vi "TcA04-002_ForceParentCallMethods.vi"(1 "Input buffer":T3="1", 3 "Invocation info":T2, 5 "error in (no error)":errorcluster, 6 "Add log to result?":bool) -> (16 "Test Data":T1 {"Numeric Measurement" format="%.2f"}, 19 "error out":errorcluster)   [LabVIEW 2020]
doc: "Test case template."
uses:
  Shared/Support_InputBuffer.ctl
  Shared/Support_InvocationInfo.ctl
  Shared/Support_TestData.ctl
  TestClasses/G#BaseClass1_class/G#BaseClass1.lvclass
  TestClasses/G#SubClass1_class/G#SubClass1.lvclass
  C:/Program Files (x86)/National Instruments/LabVIEW 2020/vi.lib/addons/_AddQ/G#Object/G#Object.lvclass
  TestClasses/G#SubSubClass1_class/G#SubSubClass1.lvclass
  <vilib>/addons/_AddQ/G#Object/G#Object.lvclass
panel:
  in  "Test name":string="TcA04-002 Force Parent Call Methods"
  out "Test result":bool
  out "Result":string
  # "Verify that a sub class method can be dynamically called\n(if there exists one) by a virtually declared base \nclass method else base class implementation is used."
  # "Sub test case"
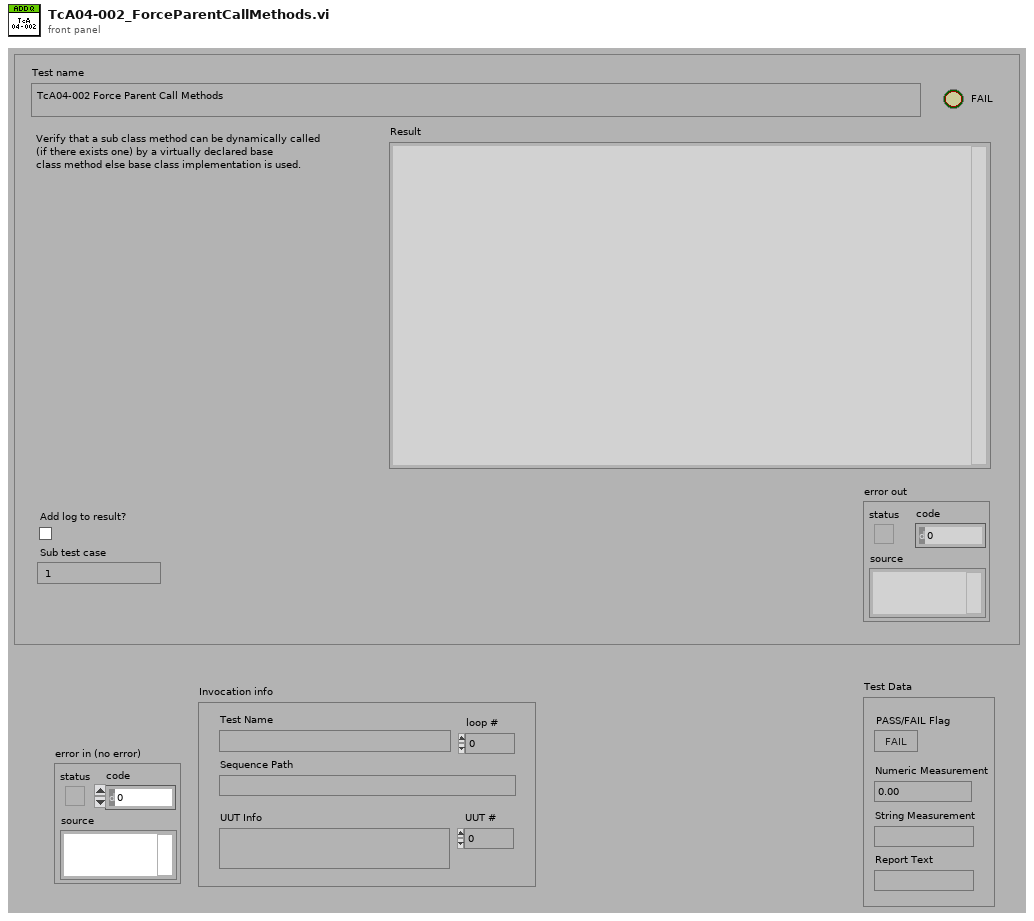
[diagram p1: front panel]
types:
  T1 = typedef "Support_TestData.ctl" = cluster{"PASS/FAIL Flag":bool, "Numeric Measurement":dbl, "String Measurement":string, "Report Text":string}
  T2 = typedef "Support_InvocationInfo.ctl" = cluster{"UUT #":i32, "loop #":i32, "UUT Info":string, "Test Name":string, "Sequence Path":path}
  T3 = typedef "Support_InputBuffer.ctl" = string
  T4 = typedef "Support_ResultType.ctl" = cluster{"Pass":bool, "Comment":string, "MeasurementValue":dbl}
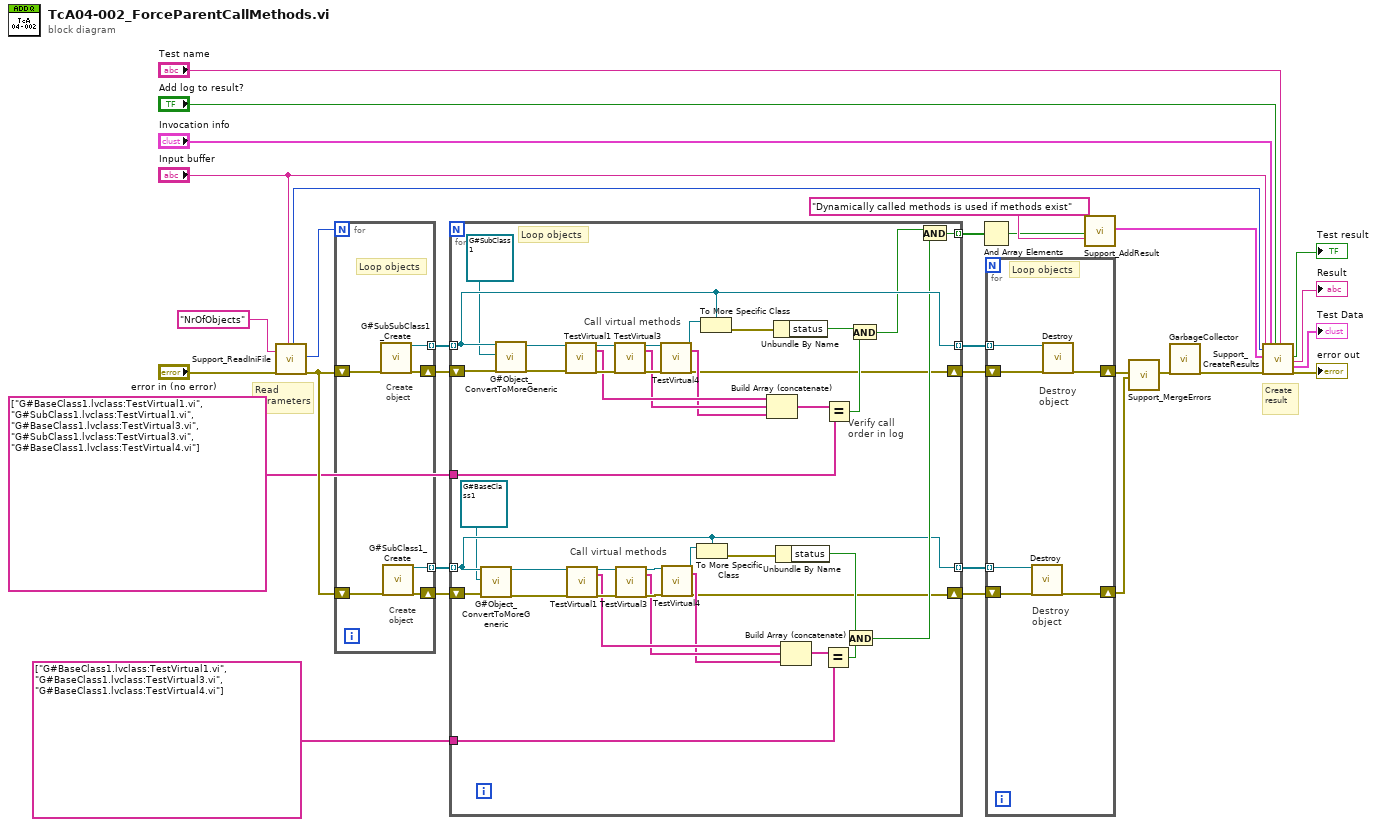
[diagram p0: block diagram]
diagram:
  # "Create\nresult"
  # "Read\nparameters"
  n1 = call "Support_ReadIniFile.vi"("Parameter name"="NrOfObjects", "error in (no error)"="error in (no error)", "Sub test case"="Input buffer") -> ("Timer start"=w21:u32, "Parameter1 as I32"=w18:i32, "error out"=w8:errorcluster)  [unwired: 9 in, 5 out]
  n2 = for {
    N: w18 -> [_]
    tunnel: [w37] -> w15 mode=indexing
    shift-right: [w36] -> w16
    shift-left: w8 -> [w35]
    shift-right: [w33] -> w6
    shift-left: w8 -> [w34]
    tunnel: [w32] -> w7 mode=indexing
    # "Create\nobject"
    # "Loop objects"
    # "Create\nobject"
    n3 = call "G#SubSubClass1_Create.vi"("error in (no error)"=w35) -> ("reference out"=w37:refnum<class "G#SubSubClass1.lvclass">, "error out"=w36:errorcluster)  [unwired: 17 in]
    n4 = call "G#SubClass1_Create.vi"("error in (no error)"=w34) -> ("reference out"=w32:refnum<class "G#SubClass1.lvclass">, "error out"=w33:errorcluster)  [unwired: 16 in, 1 out]
  }
  n5 = for {
    shift-right: [w41] -> w14
    shift-left: w16 -> [w57]
    tunnel: w15 -> [w56] mode=indexing
    tunnel: [w56] -> w13 mode=indexing
    tunnel: [w78] -> w12 mode=indexing
    tunnel: w7 -> [w44] mode=indexing
    shift-right: [w40] -> w4
    shift-left: w6 -> [w45]
    tunnel: [w44] -> w5 mode=indexing
    tunnel: string[] ["G#BaseClass1.lvclass:TestVirtual1.vi", "G#SubClass1.lvclass:TestVirtual1.vi", "G#BaseClass1.lvclass:TestVirtual3.vi", "G#SubClass1.lvclass:TestVirtual3.vi", "G#BaseClass1.lvclass:TestVirtual4.vi"] ("appended array") -> [w60]
    tunnel: string[] ["G#BaseClass1.lvclass:TestVirtual1.vi", "G#BaseClass1.lvclass:TestVirtual3.vi", "G#BaseClass1.lvclass:TestVirtual4.vi"] ("appended array 2") -> [w58]
    # "Call virtual methods"
    # "Call virtual methods"
    # "Loop objects"
    # "Verify call\norder in log"
    n6 = call-dynamic "G#Object_ConvertToMoreGeneric.vi"("reference in"=w44, "convert to"=refnum<class "G#BaseClass1.lvclass"> refnum ("G#BaseClass1.lvclass"), "error in (no error)"=w45) -> ("converted reference out"=w42:refnum<class "G#BaseClass1.lvclass">, "error out"=w43:errorcluster)  [unwired: 15 in]
    n7 = call-dynamic "G#Object_ConvertToMoreGeneric.vi"("reference in"=w56, "convert to"=refnum<class "G#SubClass1.lvclass"> refnum ("G#SubClass1.lvclass"), "error in (no error)"=w57) -> ("converted reference out"=w54:refnum<class "G#SubClass1.lvclass">, "error out"=w55:errorcluster)  [unwired: 15 in]
    n8 = call-dynamic "TestVirtual1.vi"("reference in"=w54, "error in (no error)"=w55) -> ("reference out"=w75:refnum<class "G#SubClass1.lvclass">, "MethodName"=w67:string[], "error out"=w77:errorcluster)  [unwired: 15 in]
    n9 = call-dynamic "TestVirtual1.vi"("reference in"=w42, "error in (no error)"=w43) -> ("reference out"=w71:refnum<class "G#BaseClass1.lvclass">, "MethodName"=w63:string[], "error out"=w70:errorcluster)  [unwired: 15 in]
    n10 = call-dynamic "TestVirtual3.vi"("reference in"=w75, "error in (no error)"=w77) -> ("reference out"=w74:refnum<class "G#SubClass1.lvclass">, "MethodName"=w66:string[], "error out"=w76:errorcluster)  [unwired: 15 in]
    n11 = call-dynamic "TestVirtual3.vi"("reference in"=w71, "error in (no error)"=w70) -> ("reference out"=w72:refnum<class "G#BaseClass1.lvclass">, "MethodName"=w62:string[], "error out"=w69:errorcluster)  [unwired: 15 in]
    n12 = call-dynamic "TestVirtual4.vi"("reference in"=w74, "error in (no error)"=w76) -> ("reference out"=w73:refnum<class "G#SubClass1.lvclass">, "MethodName"=w65:string[], "error out"=w41:errorcluster)  [unwired: 15 in]
    n13 = call-dynamic "TestVirtual4.vi"("reference in"=w72, "error in (no error)"=w69) -> ("reference out"=w68:refnum<class "G#BaseClass1.lvclass">, "MethodName"=w61:string[], "error out"=w40:errorcluster)  [unwired: 15 in]
    n14 = To More Specific Class(target class=w44, reference=w68) -> (error out=w49:errorcluster)  [unwired: 1 in, 1 out]
    n15 = To More Specific Class(target class=w56, reference=w73) -> (error out=w53:errorcluster)  [unwired: 1 in, 1 out]
    n16 = Build Array (concatenate)(w67, w66, w65) -> (w64:string[])
    n17 = Unbundle By Name(w53) -> ("status"=w52:bool)
    n18 = Unbundle By Name(w49) -> ("status"=w48:bool)
    n19 = Build Array (concatenate)(w63, w62, w61) -> (w59:string[])
    n20 = Equal?(x=w59, y=w58) -> (x = y?=w47:bool)
    n21 = Equal?(x=w64, y=w60) -> (x = y?=w51:bool)
    n22 = And(x=w48, y=w47) -> (x .and. y?=w46:bool)
    n23 = And(x=w52, y=w51) -> (x .and. y?=w50:bool)
    n24 = And(x=w50, y=w46) -> (x .and. y?=w78:bool)
  }
  n25 = And Array Elements(Boolean array=w12) -> (logical AND=w11:bool)
  n26 = for {
    shift-right: [w84] -> w9
    shift-left: w14 -> [w83]
    tunnel: w13 -> [w82] mode=indexing
    tunnel: w5 -> [w81] mode=indexing
    shift-right: [w79] -> w3
    shift-left: w4 -> [w80]
    # "Destroy\nobject"
    # "Loop objects"
    # "Destroy\nobject"
    n27 = call-dynamic "Destroy.vi"("reference in"=w81, "error in (no error)"=w80) -> ("error out"=w79:errorcluster)  [unwired: 16 in, 1 out]
    n28 = call-dynamic "Destroy.vi"("reference in"=w82, "error in (no error)"=w83) -> ("error out"=w84:errorcluster)  [unwired: 16 in, 1 out]
  }
  n29 = call "Support_AddResult.vi"("Pass"=w11, "Comment"="Dynamically called methods is used if methods exist") -> ("Results out"=w24:T4[])  [unwired: 17 in]
  n30 = call "Support_MergeErrors.vi"("error in 1"=w9, "error in 2"=w3) -> ("error out"=w10:errorcluster)  [unwired: 16 in, 1 out]
  n31 = call <vilib>:"GarbageCollector.vi"("error in (no error)"=w10) -> ("error out"=w20:errorcluster)  [unwired: 16 in, 2 out]
  n32 = call "Support_CreateResults.vi"("Sub test case"="Input buffer", "Timer start"=w21, "Results"=w24, "error in (no error)"=w20, "Invocation info"="Invocation info", "Add log to result?"="Add log to result?", "Test name"="Test name") -> ("Pass/fail flag"=→"Test result":bool, "Result"=→"Result":string, "Test Data"=→"Test Data":T1, "error out"=→"error out":errorcluster)  [unwired: 9 in]
